vi "SendFLCam_DAC.vi"(6 "feature":u8, 7 "data":u16, 8 "error in (no error)":errorcluster, 9 "addr":u8, 10 "ctrl":u8) -> (0 "error out":errorcluster)   [LabVIEW 2015, in "ESLSCDLL.lvlib"]
uses:
  ESLSCDLL.lvlib
  Globals.vi
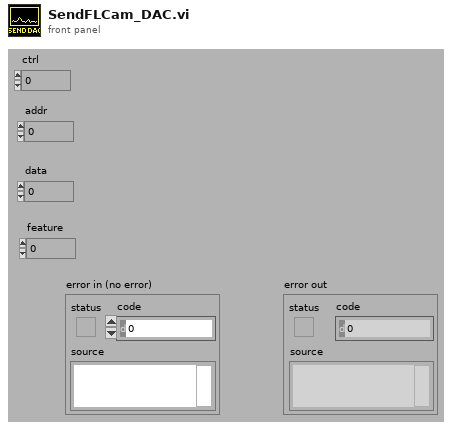
[diagram p1: front panel]
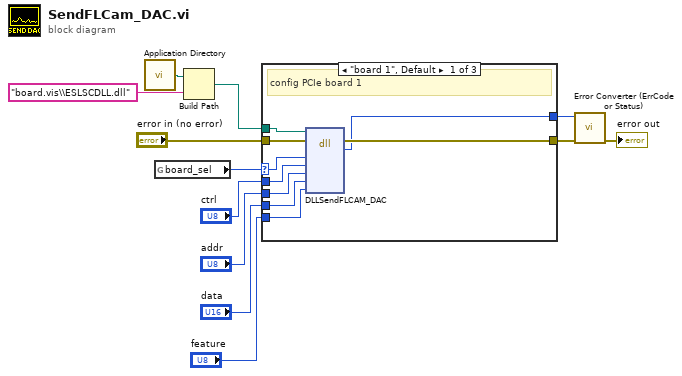
[diagram p0: block diagram]
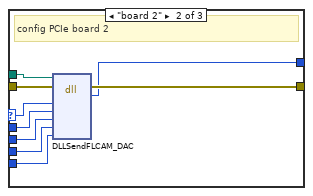
[diagram p2: hidden frame]
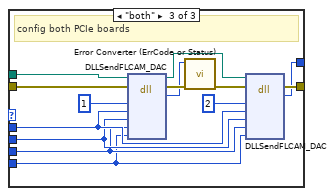
[diagram p3: hidden frame]
diagram:
  n1 = call <vilib>:"Application Directory.vi"() -> ("Application Directory"=w3:path)
  n2 = global read "Globals.vi" "board_sel"() -> (w4:enum32{"0", "board 1", "board 2", "both"})
  n3 = Build Path(base path=w3, name or relative path="board.vis\\ESLSCDLL.dll") -> (appended path=w1:path)
  n4 = case shown="\"board 1\", Default" w4 {
    selector: w4 -> [w21 w26 _]
    tunnel: "feature" -> [w20 w27 w39]
    tunnel: "data" -> [w19 w28 w40]
    tunnel: "addr" -> [w18 w29 w41]
    tunnel: "ctrl" -> [w17 w30 w42]
    tunnel: "error in (no error)" -> [w16 w25 w33]
    tunnel: [w15 w24 w35] -> w6
    tunnel: [w14 w23 w34] -> w5
    tunnel: w1 -> [w13 w22 w32]
    frame "board 1", Default {
      # "config PCIe board 1"
      n5 = dll-call lib="C:/ENTW/PCIE/LV64/board.vis/ESLSCDLL.dll" fn="DLLSendFLCAM_DAC" ("lwlscdll.dll:DLLSetADAmpRed")(path in=w13, error in=w16, "drvno"=w21, "ctrl"=w17, "addr"=w18, "data"=w19, "feature"=w20) -> (error out=w15:errorcluster, "es_status_codes"=w14:i32)  [unwired: 6 in, 1 out]
    }
    frame "board 2" {
      # "config PCIe board 2"
      n6 = dll-call lib="C:/ENTW/PCIE/LV64/board.vis/ESLSCDLL.dll" fn="DLLSendFLCAM_DAC" ("lwlscdll.dll:DLLSetADAmpRed")(path in=w22, error in=w25, "drvno"=w26, "ctrl"=w30, "addr"=w29, "data"=w28, "feature"=w27) -> (error out=w24:errorcluster, "es_status_codes"=w23:i32)  [unwired: 6 in, 1 out]
    }
    frame "both" {
      # "config both PCIe boards"
      n7 = dll-call lib="C:/ENTW/PCIE/LV64/board.vis/ESLSCDLL.dll" fn="DLLSendFLCAM_DAC" ("lwlscdll.dll:DLLSetADAmpRed")(path in=w32, error in=w33, "drvno"=u32 1, "ctrl"=w42, "addr"=w41, "data"=w40, "feature"=w39) -> (path out=w31:path, error out=w38:errorcluster, "es_status_codes"=w37:i32)  [unwired: 6 in]
      n8 = call "Error Converter (ErrCode or Status).vi"("error in (no error)"=w38, "error code"=w37) -> ("error out"=w36:errorcluster)  [unwired: 9 in]
      n9 = dll-call lib="C:/ENTW/PCIE/LV64/board.vis/ESLSCDLL.dll" fn="DLLSendFLCAM_DAC" ("lwlscdll.dll:DLLSetADAmpRed")(path in=w31, error in=w36, "drvno"=u32 2, "ctrl"=w42, "addr"=w41, "data"=w40, "feature"=w39) -> (error out=w35:errorcluster, "es_status_codes"=w34:i32)  [unwired: 6 in, 1 out]
    }
  }
  n10 = call "Error Converter (ErrCode or Status).vi"("error in (no error)"=w6, "error code"=w5) -> ("error out"=→"error out":errorcluster)  [unwired: 9 in]
